vi "Teleop Arm and Shoot.vi"(11 "Joystick Data":T1) -> ()   [LabVIEW 2013]
uses:
  Joystick Data.ctl
  Shooter state.ctl
  <vilib>/Rock Robotics/WPI/Solenoid/WPI_SolenoidValue.ctl
  Robot Global Data.vi
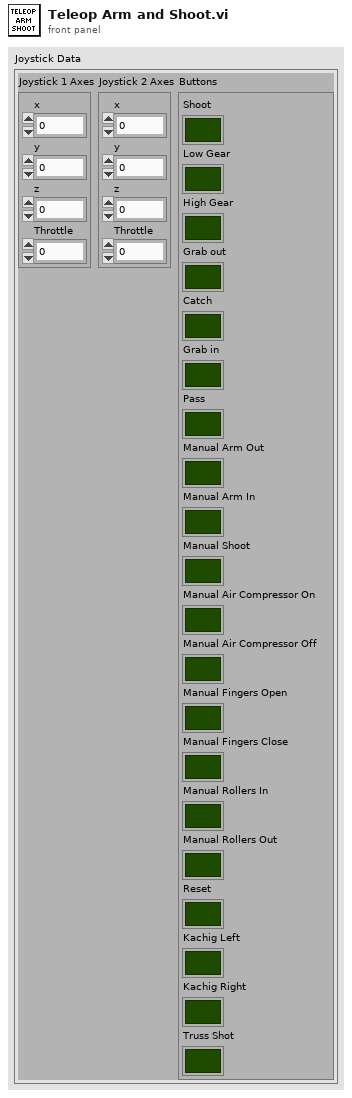
[diagram p1: front panel]
types:
  T1 = typedef "Joystick Data.ctl" = cluster{"Joystick 1 Axes":cluster{"x":dbl, "y":dbl, "z":dbl, "Throttle":dbl}, "Joystick 2 Axes":cluster{"x":dbl, "y":dbl, "z":dbl, "Throttle":dbl}, "Buttons":cluster{"Shoot":bool, "Low Gear":bool, "High Gear":bool, "Grab out":bool, "Catch":bool, "Grab in":bool, "Pass":bool, "Manual Arm Out":bool, "Manual Arm In":bool, "Manual Shoot":bool, "Manual Air Compressor On":bool, "Manual Air Compressor Off":bool, "Manual Fingers Open":bool, "Manual Fingers Close":bool, "Manual Rollers In":bool, "Manual Rollers Out":bool, "Reset":bool, "Kachig Left":bool, "Kachig Right":bool, "Truss Shot":bool}}
  T2 = typedef "WPI_DigitalInputDevRef.ctl" = cluster{"DevStatus":errorcluster, "DIO Channel":T3, "Digital Module":T4}
  T3 = typedef "FPGA_DIOChannel.ctl" = enum8{"DIO 1", "DIO 2", "DIO 3", "DIO 4", "DIO 5", "DIO 6", "DIO 7", "DIO 8", "DIO 9", "DIO 10", "DIO 11", "DIO 12", "DIO 13", "DIO 14", "Invalid"}
  T4 = typedef "FPGA_TypedefDigitalModule.ctl" = enum16{"Digital Module 1", "Digital Module 2"}
  T5 = typedef "Shooter state.ctl" = enum16{"idle", "shoot", "pass", "grab out", "grab in", "reset", "catch", "truss"}
  T6 = typedef "WPI_SolenoidValue.ctl" = enum16{"Off", "On", "Forward", "Reverse"}
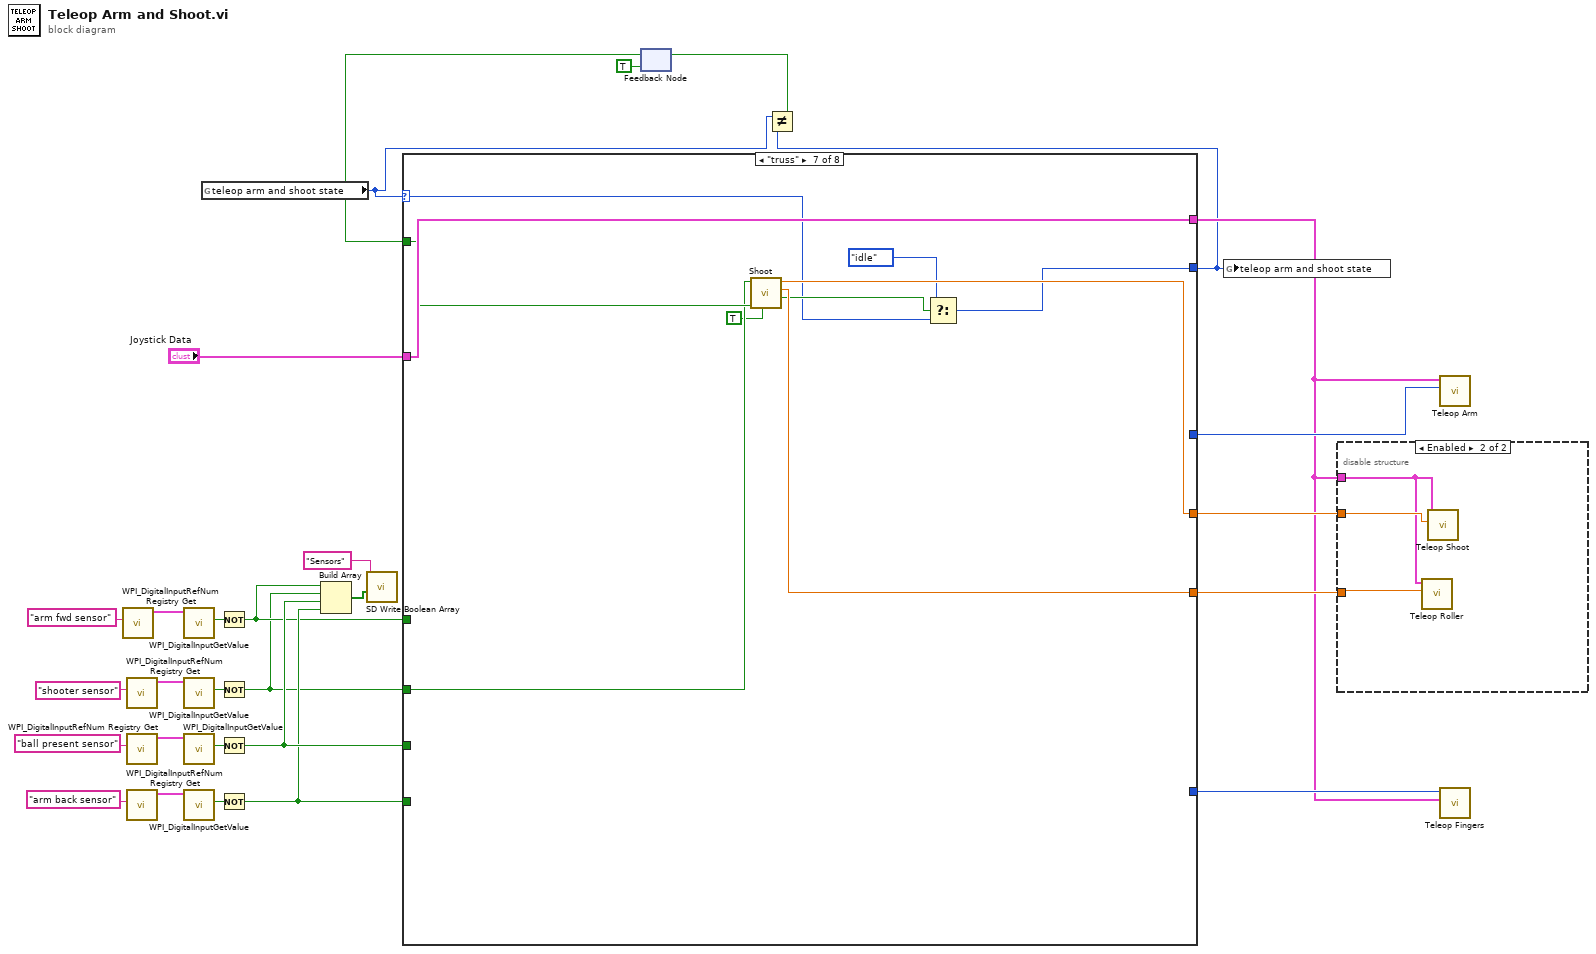
[diagram p0: block diagram]
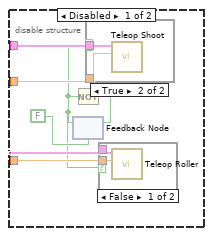
[diagram p2: hidden frame]
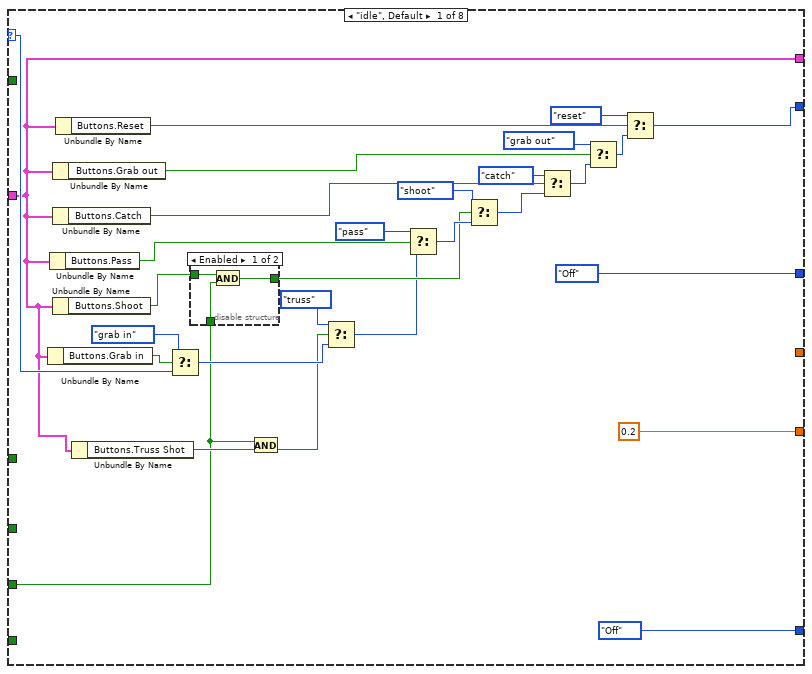
[diagram p5: hidden frame]
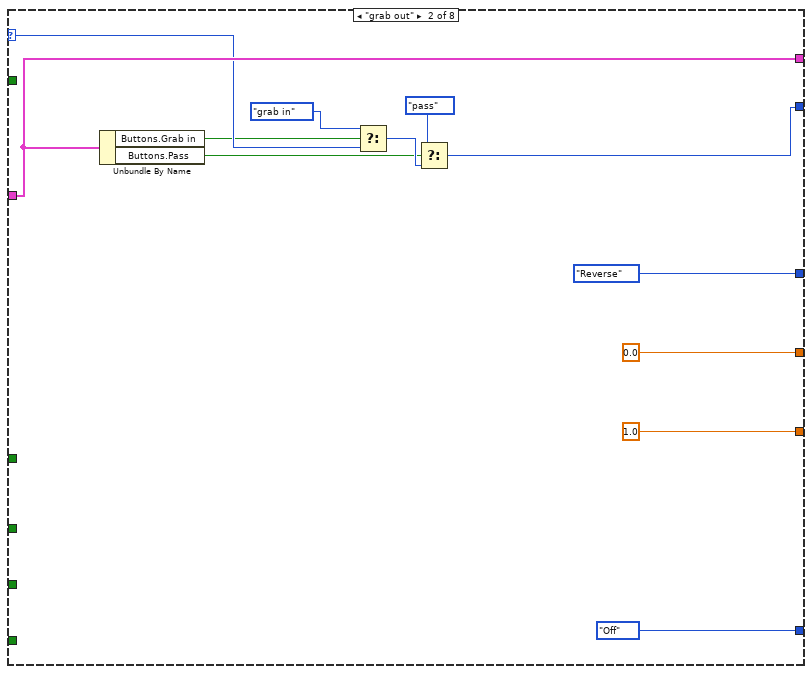
[diagram p7: hidden frame]
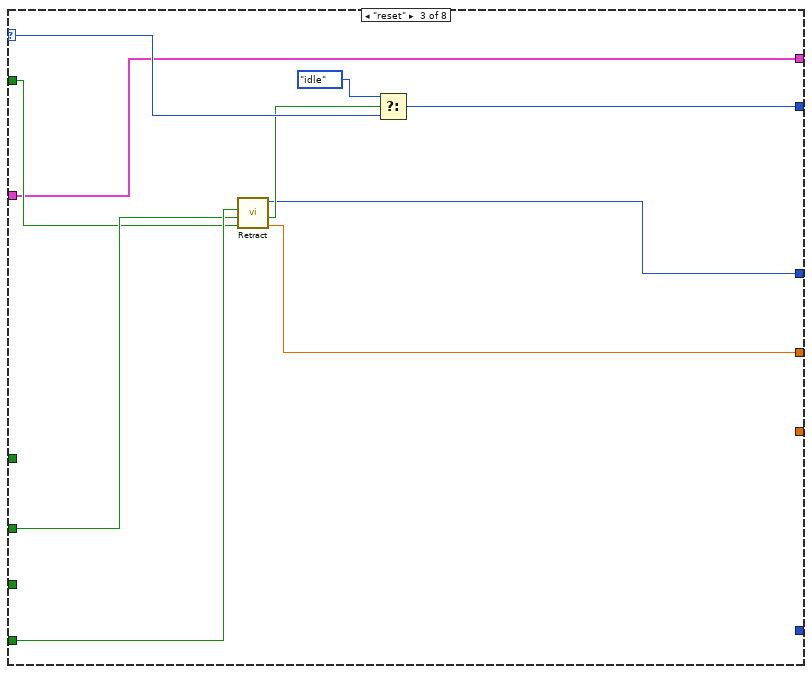
[diagram p8: hidden frame]
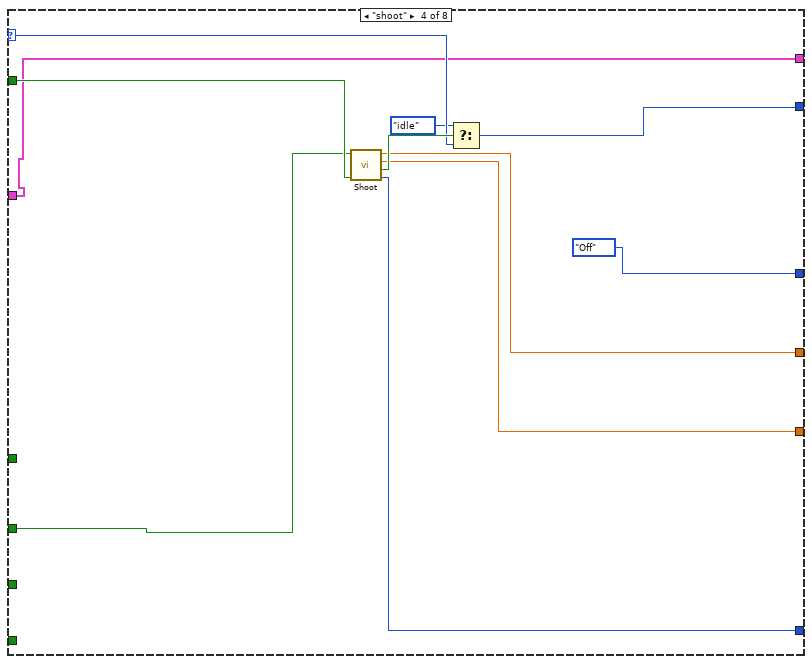
[diagram p9: hidden frame]
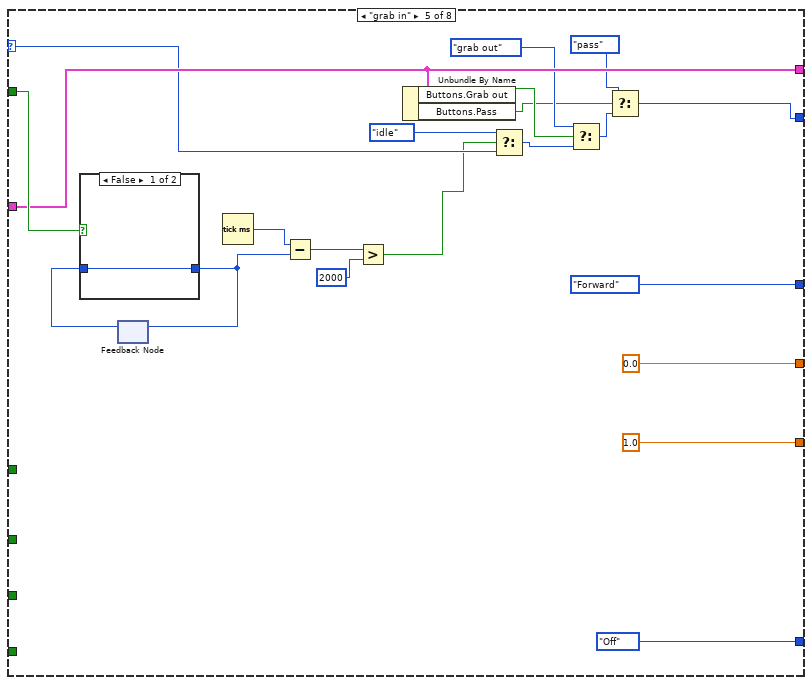
[diagram p10: hidden frame]
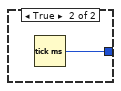
[diagram p11: hidden frame]
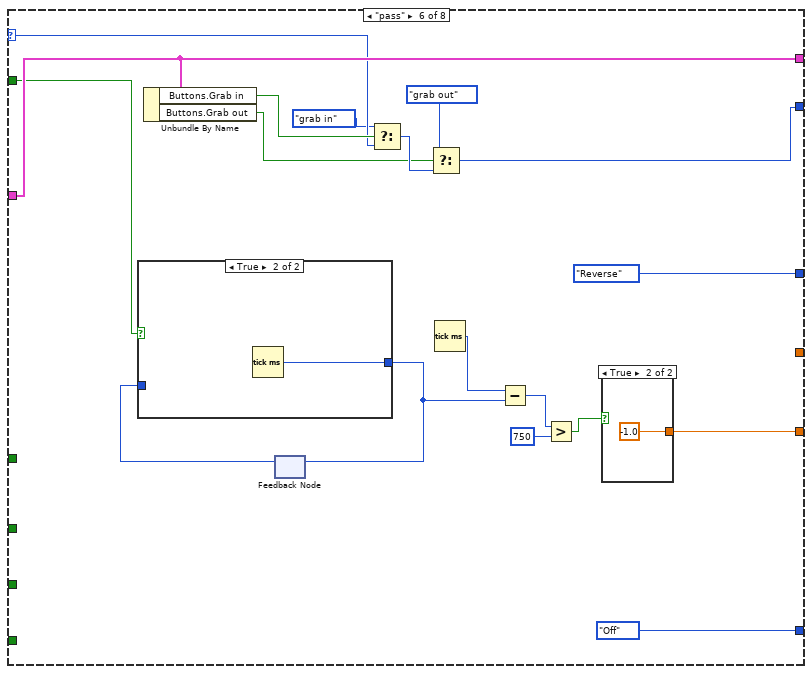
[diagram p12: hidden frame]
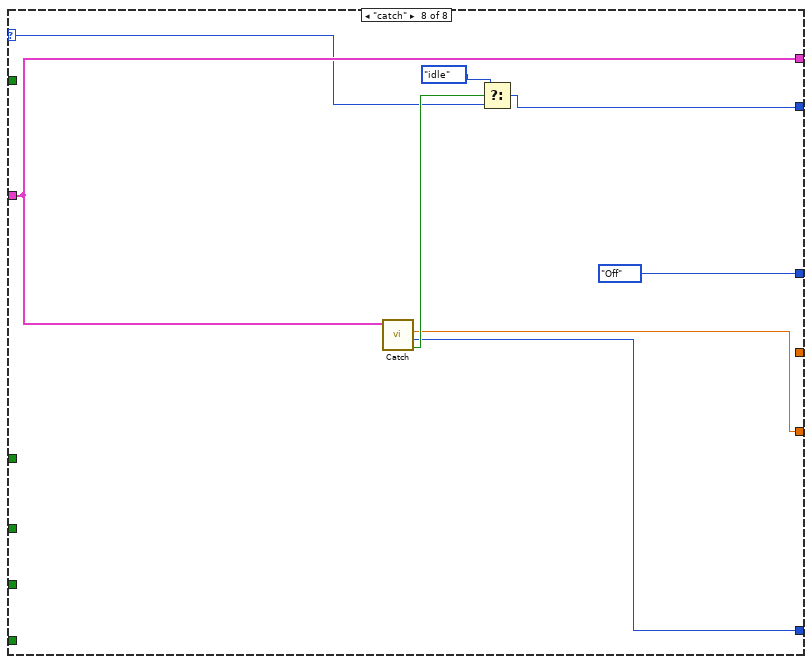
[diagram p15: hidden frame]
diagram:
  n1 = call <vilib>:"WPI_DigitalInputRefNum Registry Get.vi"("refnum name"="arm fwd sensor") -> ("DigitalInputDevRef"=w24:T2)  [unwired: 9 in, 1 out]
  n2 = call <vilib>:"WPI_DigitalInputRefNum Registry Get.vi"("refnum name"="shooter sensor") -> ("DigitalInputDevRef"=w16:T2)  [unwired: 9 in, 1 out]
  n3 = call <vilib>:"WPI_DigitalInputRefNum Registry Get.vi"("refnum name"="ball present sensor") -> ("DigitalInputDevRef"=w19:T2)  [unwired: 9 in, 1 out]
  n4 = call <vilib>:"WPI_DigitalInputRefNum Registry Get.vi"("refnum name"="arm back sensor") -> ("DigitalInputDevRef"=w5:T2)  [unwired: 9 in, 1 out]
  n5 = call <vilib>:"WPI_DigitalInputGetValue.vi"("DigitalInputDevRef"=w24) -> ("Value"=w20:bool)  [unwired: 8 in, 2 out]
  n6 = call <vilib>:"WPI_DigitalInputGetValue.vi"("DigitalInputDevRef"=w16) -> ("Value"=w21:bool)  [unwired: 8 in, 2 out]
  n7 = call <vilib>:"WPI_DigitalInputGetValue.vi"("DigitalInputDevRef"=w19) -> ("Value"=w22:bool)  [unwired: 8 in, 2 out]
  n8 = call <vilib>:"WPI_DigitalInputGetValue.vi"("DigitalInputDevRef"=w5) -> ("Value"=w4:bool)  [unwired: 8 in, 2 out]
  n9 = global read "Robot Global Data.vi" "teleop arm and shoot state"() -> (w2:T5)
  n10 = Not(x=w20) -> (.not. x?=w27:bool)
  n11 = Not(x=w21) -> (.not. x?=w26:bool)
  n12 = Not(x=w22) -> (.not. x?=w29:bool)
  n13 = Not(x=w4) -> (.not. x?=w28:bool)
  n14 = Build Array(w27, w26, w29, w28) -> (w14:bool[])
  n15 = call <vilib>:"SD Write Boolean Array.vi"("Boolean Array"=w14, "Name"="Sensors") -> ()  [unwired: 8 in, 2 out]
  n16 = feedback #1(TRUE) -> (w8:bool)
  n17 = case shown="\"truss\"" w2 {
    selector: w2 -> [w39 w68 w84 w94 w98 w132 w143 w155]
    tunnel: w26 -> [_ _ w79 w85 _ _ w145 _]
    tunnel: w29 -> [w30 _ _ _ _ _ _ _]
    tunnel: w28 -> [_ _ w80 _ _ _ _ _]
    tunnel: [w37 w64 w76 w86 w101 w126 w141 w153] -> w1
    tunnel: [0.2 ("Roller Speed") 1.0 ("Roller Speed") _ w91 1.0 ("Roller Speed") w135 w148 w152] -> w10
    tunnel: [_ 0.0 ("shooter speed") w81 w92 0.0 ("shooter speed") _ w147 _] -> w11
    tunnel: [WPI_SolenoidValue."Off" ("Arm Out") WPI_SolenoidValue."Reverse" ("Arm State") w75 WPI_SolenoidValue."Off" ("Arm State") WPI_SolenoidValue."Forward" ("Arm State") WPI_SolenoidValue."Reverse" ("Arm State") _ WPI_SolenoidValue."Off" ("Arm State")] -> w12
    tunnel: w27 -> [_ _ _ _ _ _ _ _]
    tunnel: w8 -> [_ _ w78 w90 w114 w124 w146 _]
    tunnel: [WPI_SolenoidValue."Off" ("Pivot state") WPI_SolenoidValue."Off" ("Pivot state") _ w89 WPI_SolenoidValue."Off" ("Pivot state") WPI_SolenoidValue."Off" ("Pivot state") _ w151] -> w13
    tunnel: "Joystick Data" -> [w35 w70 w77 w88 w106 w134 w149 w157]
    tunnel: [w35 w70 w77 w88 w106 w134 w149 w157] -> w9
    frame "idle", Default {
      n18 = Unbundle By Name(w35) -> ("Buttons.Grab in"=w40:bool)
      n19 = Unbundle By Name(w35) -> ("Buttons.Pass"=w43:bool)
      n20 = Unbundle By Name(w35) -> ("Buttons.Grab out"=w47:bool)
      n21 = Unbundle By Name(w35) -> ("Buttons.Catch"=w50:bool)
      n22 = Unbundle By Name(w35) -> ("Buttons.Shoot"=w42:bool)
      n23 = Unbundle By Name(w35) -> ("Buttons.Reset"=w48:bool)
      n24 = Unbundle By Name(w35) -> ("Buttons.Truss Shot"=w36:bool)
      n25 = Select(t=Shooter_state."grab in", s=w40, f=w39) -> (s? t:f=w33:T5)
      n26 = disable-structure shown="Enabled" {
        disable-tunnel: [w61 w62] -> w56
        disable-tunnel: w30 -> [w60 _]
        disable-tunnel: w42 -> [w59 w62]
        frame Enabled {
          n27 = And(x=w59, y=w60) -> (x .and. y?=w61:bool)
        }
        frame Disabled {
        }
      }
      n28 = And(x=w30, y=w36) -> (x .and. y?=w31:bool)
      n29 = Select(t=Shooter_state."truss", s=w31, f=w33) -> (s? t:f=w32:T5)
      n30 = Select(t=Shooter_state."pass", s=w43, f=w32) -> (s? t:f=w58:T5)
      n31 = Select(t=Shooter_state."shoot", s=w56, f=w58) -> (s? t:f=w52:T5)
      n32 = Select(t=Shooter_state."catch", s=w50, f=w52) -> (s? t:f=w46:T5)
      n33 = Select(t=Shooter_state."grab out", s=w47, f=w46) -> (s? t:f=w49:T5)
      n34 = Select(t=Shooter_state."reset", s=w48, f=w49) -> (s? t:f=w37:T5)
    }
    frame "grab out" {
      n35 = Unbundle By Name(w70) -> ("Buttons.Grab in"=w67:bool, "Buttons.Pass"=w63:bool)
      n36 = Select(t=Shooter_state."grab in", s=w67, f=w68) -> (s? t:f=w66:T5)
      n37 = Select(t=Shooter_state."pass", s=w63, f=w66) -> (s? t:f=w64:T5)
    }
    frame "reset" {
      n38 = call "Retract.vi"("Reset"=w78, "Shooter Sensor"=w79, "Arm Up Sensor"=w80) -> ("Shooter Motor"=w81:dbl, "Finished"=w82:bool, "Arm"=w75:T6)  [unwired: 6 in]
      n39 = Select(t=Shooter_state."idle", s=w82, f=w84) -> (s? t:f=w76:T5)
    }
    frame "shoot" {
      n40 = call "Shoot.vi"("Reset"=w90, "Shooter Sensor"=w85) -> ("Arm fingers state"=w89:T6, "Finished?"=w95:bool, "Roller Motor Value"=w91:dbl, "Shooter Motor Value"=w92:dbl)  [unwired: 6 in]
      n41 = Select(t=Shooter_state."idle", s=w95, f=w94) -> (s? t:f=w86:T5)
    }
    frame "grab in" {
      n42 = feedback #2() -> (w113:u32)  [unwired: 1 in]
      n43 = case shown="False" w114 {
        tunnel: [w117 w118] -> w111
        tunnel: w113 -> [w117 _]
        frame False {
        }
        frame True {
          n44 = Tick Count (ms)() -> (millisecond timer value=w118:u32)
        }
      }
      n45 = feedback-in #2(w111) -> ()
      n46 = Tick Count (ms)() -> (millisecond timer value=w112:u32)
      n47 = Subtract(x=w112, y=w111) -> (x-y=w110:u32)
      n48 = Greater?(x=w110, y=u32 2000) -> (0:w96:bool)
      n49 = Unbundle By Name(w106) -> ("Buttons.Grab out"=w104:bool, "Buttons.Pass"=w100:bool)
      n50 = Select(t=Shooter_state."idle", s=w96, f=w98) -> (s? t:f=w105:T5)
      n51 = Select(t=Shooter_state."grab out", s=w104, f=w105) -> (s? t:f=w102:T5)
      n52 = Select(t=Shooter_state."pass", s=w100, f=w102) -> (s? t:f=w101:T5)
    }
    frame "pass" {
      n53 = Unbundle By Name(w134) -> ("Buttons.Grab in"=w133:bool, "Buttons.Grab out"=w128:bool)
      n54 = feedback #3() -> (w125:u32)  [unwired: 1 in]
      n55 = case shown="True" w124 {
        tunnel: w125 -> [w138 _]
        tunnel: [w138 w139] -> w122
        frame False {
        }
        frame True {
          n56 = Tick Count (ms)() -> (millisecond timer value=w139:u32)
        }
      }
      n57 = feedback-in #3(w122) -> ()
      n58 = Select(t=Shooter_state."grab in", s=w133, f=w132) -> (s? t:f=w129:T5)
      n59 = Select(t=Shooter_state."grab out", s=w128, f=w129) -> (s? t:f=w126:T5)
      n60 = Tick Count (ms)() -> (millisecond timer value=w123:u32)
      n61 = Subtract(x=w123, y=w122) -> (x-y=w121:u32)
      n62 = Greater?(x=w121, y=u32 750) -> (0:w120:bool)
      n63 = case shown="True" w120 {
        tunnel: [_ -1.0 ("Roller Speed")] -> w135
        frame False {
        }
        frame True {
        }
      }
    }
    frame "truss" {
      n64 = call "Shoot.vi"("Truss?"=TRUE, "Reset"=w146, "Shooter Sensor"=w145) -> ("Finished?"=w144:bool, "Roller Motor Value"=w148:dbl, "Shooter Motor Value"=w147:dbl)  [unwired: 5 in, 1 out]
      n65 = Select(t=Shooter_state."idle", s=w144, f=w143) -> (s? t:f=w141:T5)
    }
    frame "catch" {
      n66 = call "Catch.vi"("Joystick Data"=w157) -> ("Finished"=w156:bool, "Arm finger state"=w151:T6, "Roller Speed"=w152:dbl)  [unwired: 8 in]
      n67 = Select(t=Shooter_state."idle", s=w156, f=w155) -> (s? t:f=w153:T5)
    }
  }
  n68 = Not Equal?(x=w2, y=w1) -> (x != y?=w3:bool)
  n69 = feedback-in #1(w3) -> ()
  n70 = global write "Robot Global Data.vi" "teleop arm and shoot state"(w1) -> ()
  n71 = disable-structure shown="Enabled" {
    disable-tunnel: w11 -> [w163 w170]
    disable-tunnel: w10 -> [w162 w168]
    disable-tunnel: w9 -> [w161 w169]
    frame Disabled {
      n72 = feedback #4(FALSE) -> (w158:bool)
      n73 = Not(x=w158) -> (.not. x?=w159:bool)
      n74 = feedback-in #4(w159) -> ()
      n75 = case shown="True" w158 {
        tunnel: w163 -> [_ w167]
        tunnel: w161 -> [_ w166]
        frame False {
        }
        frame True {
          n76 = call "Teleop Shoot.vi"("shooter speed"=w167, "Joystick Data"=w166) -> ()  [unwired: 10 in]
        }
      }
      n77 = case shown="False" w158 {
        tunnel: w162 -> [w165 _]
        tunnel: w161 -> [w164 _]
        frame False {
          n78 = call "Teleop Roller.vi"("Roller Speed"=w165, "Joystick Data"=w164) -> ()  [unwired: 10 in]
        }
        frame True {
        }
      }
    }
    frame Enabled {
      n79 = call "Teleop Roller.vi"("Roller Speed"=w168, "Joystick Data"=w169) -> ()  [unwired: 10 in]
      n80 = call "Teleop Shoot.vi"("shooter speed"=w170, "Joystick Data"=w169) -> ()  [unwired: 10 in]
    }
  }
  n81 = call "Teleop Arm.vi"("Arm State"=w12, "Joystick Data"=w9) -> ()  [unwired: 10 in]
  n82 = call "Teleop Fingers.vi"("Joystick Data"=w9, "Arm Out"=w13) -> ()  [unwired: 10 in]
